vi "007 Crear dos arrays 100 posicions.vi"() -> ()   [LabVIEW 2019]
panel:
  out "Random temp":cluster{dbl, dbl, dbl[]}[](graph)
  in  "TempMax":i32
  in  "TempMin":i32
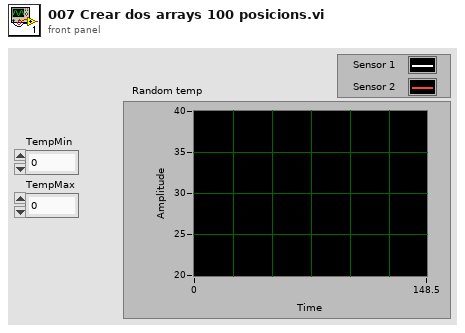
[diagram p1: front panel]
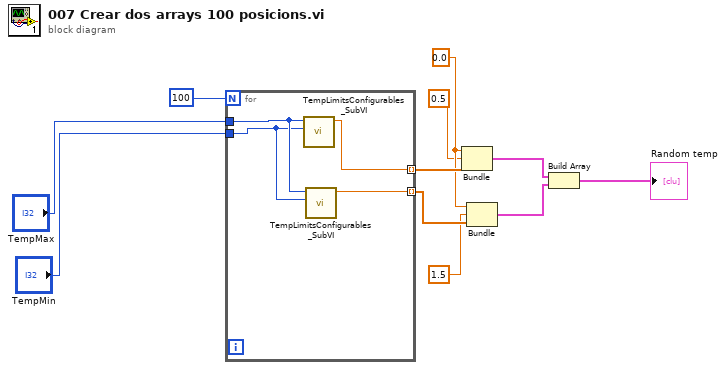
[diagram p0: block diagram]
diagram:
  w3 = 0.0
  n1 = for {
    N: 100 -> [_]
    tunnel: "TempMax" -> [w15]
    tunnel: "TempMin" -> [w14]
    tunnel: [w13] -> w7 mode=indexing
    tunnel: [w12] -> w8 mode=indexing
    n2 = call "TempLimitsConfigurables_SubVI.vi"("TempMin"=w14, "TempMax"=w15) -> ("RandomTemp"=w12:dbl)  [unwired: 9 in]
    n3 = call "TempLimitsConfigurables_SubVI.vi"("TempMin"=w14, "TempMax"=w15) -> ("RandomTemp"=w13:dbl)  [unwired: 9 in]
  }
  n4 = Bundle(w3, 0.5, w8) -> (w6:cluster{dbl, dbl, dbl[]})  [unwired: 1 in]
  n5 = Bundle(w3, 1.5, w7) -> (w5:cluster{dbl, dbl, dbl[]})  [unwired: 1 in]
  n6 = Build Array(w6, w5) -> (→"Random temp":cluster{dbl, dbl, dbl[]}[])
